vi "RWwrapper_BK.vi"(0 "Strings in":string[](array[string])=["C:\\CuspControl\\GPIB and Network\\Cusp\\RWparams.txt", "6723"], 1 "Dubs in":dbl[](array[numeric])=[1.0, 50.0, 0.05, 32.0]) -> ()   [LabVIEW 2018]
panel:
  in  "RW phase difference (degrees)":dbl=32.0
  in  "RW ON":dbl=1.0
  in  "RW amplitude (V)":dbl=0.05
  in  "RW frequency (Hz)":dbl=50.0
  in  "subvi":bool=TRUE
  in  "RW File":path=path "C:/CuspControl/GPIB and Network/Cusp/RWparams.txt"
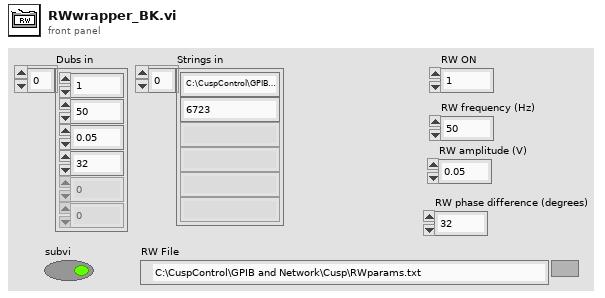
[diagram p1: front panel]
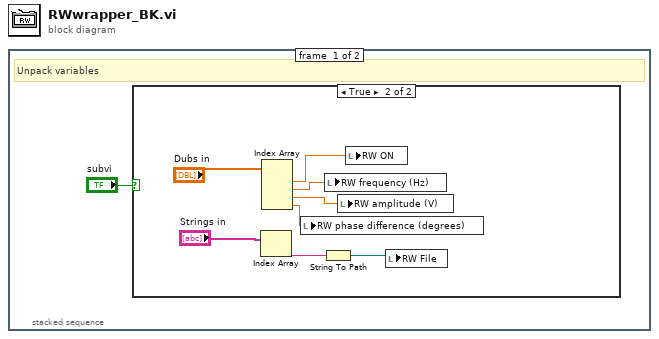
[diagram p0: block diagram]
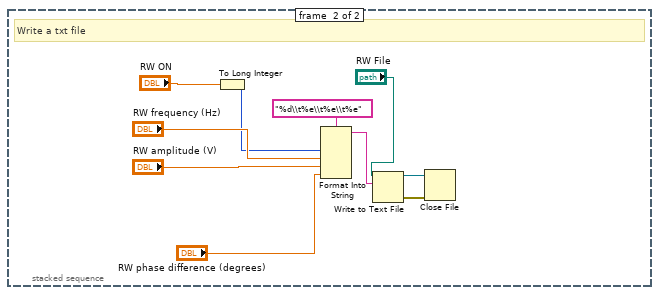
[diagram p3: hidden frame]
diagram:
  n1 = stacked-sequence {
    frame #0 {
      # "Unpack variables"
      n2 = case shown="True" "subvi" {
        frame False {
        }
        frame True {
          n3 = Index Array(array="Strings in") -> (element=w7:string)  [unwired: 1 in]
          n4 = Index Array(array="Dubs in") -> (element #1=w2:dbl, element #2=w5:dbl, element #3=w4:dbl, element #4=w3:dbl)  [unwired: 4 in]
          n5 = local write "RW phase difference (degrees)"(w3) -> ()
          n6 = String To Path(string=w7) -> (path=w6:path)
          n7 = local write "RW frequency (Hz)"(w5) -> ()
          n8 = local write "RW amplitude (V)"(w4) -> ()
          n9 = local write "RW ON"(w2) -> ()
          n10 = local write "RW File"(w6) -> ()
        }
      }
    }
    frame #1 {
      # "Write a txt file"
      n11 = To Long Integer(number="RW ON") -> (32bit integer=w12:i32)
      n12 = Format Into String(format string="%d\\t%e\\t%e\\t%e", w12, "RW frequency (Hz)", "RW amplitude (V)", "RW phase difference (degrees)") -> (resulting string=w19:string)  [unwired: 2 in, 1 out]
      n13 = Write to Text File(file (use dialog)="RW File", text=w19) -> (refnum out=w18:refnum<file>, error out=w10:errorcluster)  [unwired: 2 in, 1 out]
      n14 = Close File(refnum=w18, error in=w10) -> ()  [unwired: 2 out]
    }
  }
